vi "Read Scaling coefficients.vi"(8 "error in (no error)":errorcluster, 11 "NI-Scope Lock-in Driver in":refnum<class "NI-Scope Lock-in Driver.lvclass">) -> (0 "error out":errorcluster, 2 "Scaling coefficients":dbl[][](array[numeric]), 3 "NI-Scope Lock-in Driver out":refnum<class "NI-Scope Lock-in Driver.lvclass">)   [LabVIEW 2016, in "NI-Scope Lock-in Driver.lvclass"]
uses:
  NI-Scope Lock-in Driver.lvclass
  NI-Scope Digitizer/Ni-Scope Digitizer.lvclass
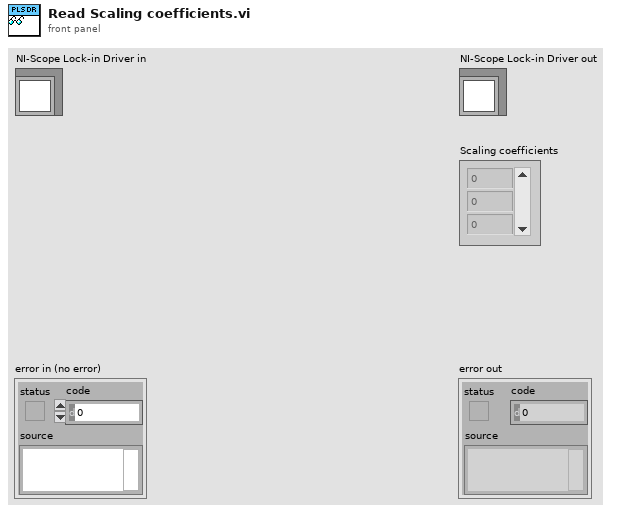
[diagram p1: front panel]
types:
  T1 = typedef "NI-Scope Lock-in Configuration.ctl" = cluster{"Points per sine wave":i32, "Rate":dbl, "Re-name channels":string[], "Active channels":string, "Ranges":dbl[], "Sync on trigger":bool, "R-Q":bool}
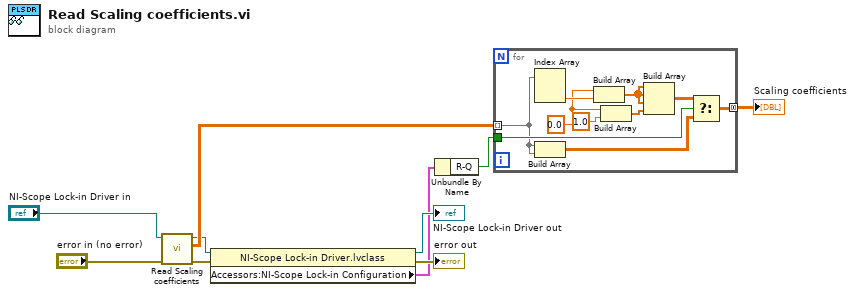
[diagram p0: block diagram]
diagram:
  n1 = call-parent "Read Scaling coefficients.vi"("error in (no error)"="error in (no error)", "Pulse Driver in"="NI-Scope Lock-in Driver in") -> ("error out"=w10:errorcluster, "Scaling coefficients"=w7:dbl[][], "Pulse Driver out"=w4:refnum<class "NI-Scope Lock-in Driver.lvclass">)  [unwired: 7 in]
  n2 = property class="NI-Scope Lock-in Driver.lvclass"(reference=w4, error in=w10) -> (reference out=→"NI-Scope Lock-in Driver out":refnum<class "NI-Scope Lock-in Driver.lvclass">, error out=→"error out":errorcluster, "Accessors:NI-Scope Lock-in Configuration"=w2:T1)
  n3 = Unbundle By Name(w2) -> ("R-Q"=w1:bool)
  n4 = for {
    tunnel: w7 -> [w14] mode=indexing
    tunnel: [w18] -> w6 mode=concatenating
    tunnel: w1 -> [w20]
    w12 = 0.0 ("element")
    n5 = Index Array(array=w14) -> (element #2=w13:dbl)  [unwired: 2 in, 1 out]
    n6 = Build Array(w14, w14) -> (w17:dbl[][])
    n7 = Build Array(w12, w13) -> (w11:dbl[])
    n8 = Build Array(w12, 1.0 ("element")) -> (w15:dbl[])
    n9 = Build Array(w11, w11, w11, w15) -> (w19:dbl[][])
    n10 = Select(t=w19, s=w20, f=w17) -> (s? t:f=w18:dbl[][])
  }
  "Scaling coefficients" <- w6
